vi "CompleteRequest.vi"(7 "Room":i32, 8 "error in (no error)":errorcluster, 9 "Fullfiller PUID":string, 10 "Complete Request":bool, 11 "Request out":refnum<class "Request.lvclass">) -> (0 "error out":errorcluster)   [LabVIEW 2015]
uses:
  LVClasses/Request/Request.lvclass
  TypeDef/RoomsActionEnum.ctl
  TypeDef/RequestActionEnum.ctl
  TypeDef/PersonnelAndTime.ctl
  LVClasses/Request/Request.lvclass/Request.ctl
  TypeDef/PersonnelActions.ctl
  LVClasses/Request/Read PUID.vi
  LVClasses/Request/Read RequestID.vi
  LVClasses/Request/Read AckName.vi
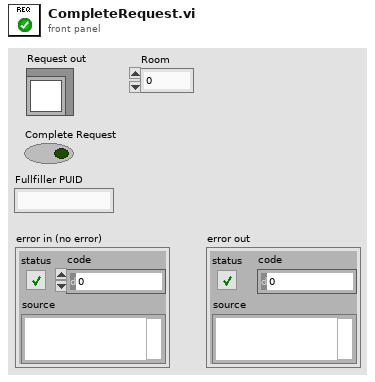
[diagram p1: front panel]
types:
  T1 = typedef "RequestActionEnum.ctl" = enum16{"Init", "ReadRequests", "ReadRequest", "AddRequest", "RemoveRequest", "ToDisk", "Ack", "Complete", "CheckAlarms", "PIntoRoom", "Read Summary", "GetRequestForRoom"}
  T2 = typedef "PersonnelAndTime.ctl" = cluster{"Personnel":string, "TimeStamp":string}
  T3 = typedef "RoomsActionEnum.ctl" = enum16{"Init", "Add Room", "Remove Room", "Read Room", "Read Flag", "Read Flag State", "Write Flag State", "Read Flag Color", "Write Flag Color", "Read Bed Vacant", "Write Bed Vacant", "Read Personnel", "Add Personnel", "Remove Personnel", "Read Requests", "Add Request", "Remove Request", "Read Beacon ID", "Write Beacon ID", "Write Bed URL", "Read Bed URL", "Read Rooms Numbers", "Write Flag"}
  T4 = typedef "PersonnelActions.ctl" = enum16{"Init", "Read Personnel", "Add Personnel", "Remove Personnel", "Read Name", "Write Name", "Read Role", "Write Role", "Read Requests", "Add Requests", "Remove Requests", "Read PUIDs", "Read PUIDs for Role", "Read All Personnel"}
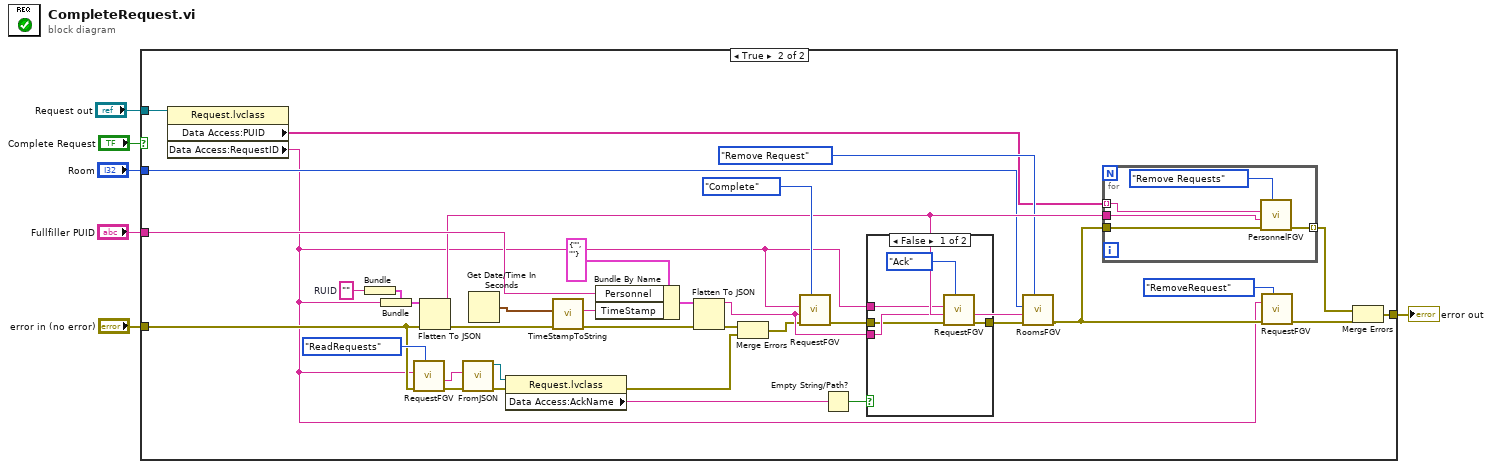
[diagram p0: block diagram]
diagram:
  n1 = case shown="True" "Complete Request" {
    tunnel: "Room" -> [_ w11]
    tunnel: "Fullfiller PUID" -> [_ w37]
    tunnel: "error in (no error)" -> [_ w23]
    tunnel: [_ w15] -> w2
    tunnel: "Request out" -> [_ w9]
    frame False {
    }
    frame True {
      w25 = ""  # RUID
      n2 = property class="Request.lvclass"(reference=w9) -> ("Data Access:PUID"=w8:string[], "Data Access:RequestID"=w7:string)  [unwired: 1 in, 2 out]
      n3 = Bundle("RUID"=w25) -> (w26:cluster{"RUID":string})  [unwired: 1 in]
      n4 = Bundle(cluster=w26, "RUID"=w7) -> (w24:cluster{"RUID":string})
      n5 = call "RequestFGV.vi"("Actions"=RequestActionEnum."ReadRequests", "error in (no error)"=w23, "RUID"=w7) -> ("error out"=w22:errorcluster, "Data Out"=w33:string)  [unwired: 7 in]
      n6 = Flatten To JSON(anything=w24, error in (no error)=w23) -> (JSON string=w12:string, 11:w27:errorcluster)  [unwired: 1 in]
      n7 = call "FromJSON.vi"("error in (no error)"=w22, "Request"=w33) -> ("error out"=w21:errorcluster, "Request out"=w32:refnum<class "Request.lvclass">)  [unwired: 8 in]
      n8 = Get Date/Time In Seconds() -> (seconds since 1Jan1904=w39:timestamp)
      n9 = property class="Request.lvclass"(reference=w32, error in=w21) -> (error out=w18:errorcluster, "Data Access:AckName"=w31:string)  [unwired: 1 out]
      n10 = call "TimeStampToString.vi"("error in (no error)"=w27, "Time Stamp"=w39) -> ("error out"=w28:errorcluster, "String"=w38:string)  [unwired: 8 in]
      n11 = Bundle By Name(cluster=T2 {"Personnel"="", "TimeStamp"=""}, "Personnel"=w37, "TimeStamp"=w38) -> (w40:T2)
      n12 = Flatten To JSON(anything=w40, error in (no error)=w28) -> (JSON string=w29:string, 11:w20:errorcluster)  [unwired: 1 in]
      n13 = Merge Errors(w20, w18) -> (w19:errorcluster)
      n14 = call "RequestFGV.vi"("Actions"=RequestActionEnum."Complete", "error in (no error)"=w19, "Data In"=w29, "RUID"=w7) -> ("error out"=w36:errorcluster)  [unwired: 6 in, 1 out]
      n15 = Empty String/Path?(string/path=w31) -> (empty?=w30:bool)
      n16 = case shown="False" w30 {
        tunnel: w7 -> [w46 _]
        tunnel: w29 -> [w45 _]
        tunnel: w36 -> [w44 w48]
        tunnel: [w43 w48] -> w14
        frame False {
          n17 = call "RequestFGV.vi"("Actions"=RequestActionEnum."Ack", "error in (no error)"=w44, "Data In"=w45, "RUID"=w46) -> ("error out"=w43:errorcluster)  [unwired: 6 in, 1 out]
        }
        frame True {
        }
      }
      n18 = call "RoomsFGV.vi"("Actions"=RoomsActionEnum."Remove Request", "error in (no error)"=w14, "Data In"=w12, "Room"=w11) -> ("error out"=w13:errorcluster)  [unwired: 6 in, 1 out]
      n19 = for {
        tunnel: w8 -> [w52] mode=indexing
        tunnel: w12 -> [w51]
        tunnel: w13 -> [w50]
        tunnel: [w49] -> w16 mode=indexing
        n20 = call "PersonnelFGV.vi"("Actions"=PersonnelActions."Remove Requests", "error in (no error)"=w50, "Data In"=w51, "PUID"=w52) -> ("error out"=w49:errorcluster)  [unwired: 6 in, 1 out]
      }
      n21 = call "RequestFGV.vi"("Actions"=RequestActionEnum."RemoveRequest", "error in (no error)"=w13, "RUID"=w7) -> ("error out"=w17:errorcluster)  [unwired: 7 in, 1 out]
      n22 = Merge Errors(w16, w17) -> (w15:errorcluster)
    }
  }
  "error out" <- w2
